vi "Read Waveform.vi"   [LabVIEW 2021, in "Yokogawa WT1800 Series.lvlib"]
doc: "Allows users to read one or more waveforms."
uses:
  <instrlib>/Yokogawa WT1800 Series/Yokogawa WT1800 Series.lvlib
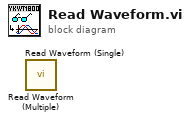
[diagram p0: block diagram]
diagram:
  n1 = call <instrlib>:"Read Waveform (Multiple).vi"() -> ()  [unwired: 9 in, 3 out]
  n2 = call <instrlib>:"Read Waveform (Single).vi"() -> ()  [unwired: 9 in, 3 out]
